vi "Motion_control_X.vi"(0 ".NET Refnum in":refnum<k24>, 1 "maxVelocity":dbl, 2 "acceleration":dbl, 3 "position":dbl) -> (7 ".NET Refnum out":refnum<k24>)   [LabVIEW 2021]
uses:
  C:/Users/User/Documents/Published_files/thorlabs_files/Thorlabs.MotionControl.IntegratedStepperMotorsCLI.dll
  thorlabs_files/Thorlabs.MotionControl.IntegratedStepperMotorsCLI.dll
panel:
  out "end":bool=TRUE
  out "x < y?":bool
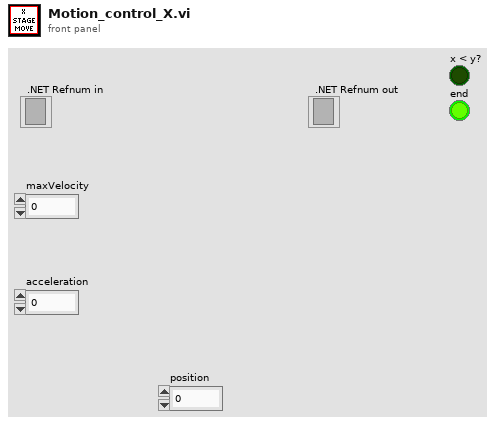
[diagram p1: front panel]
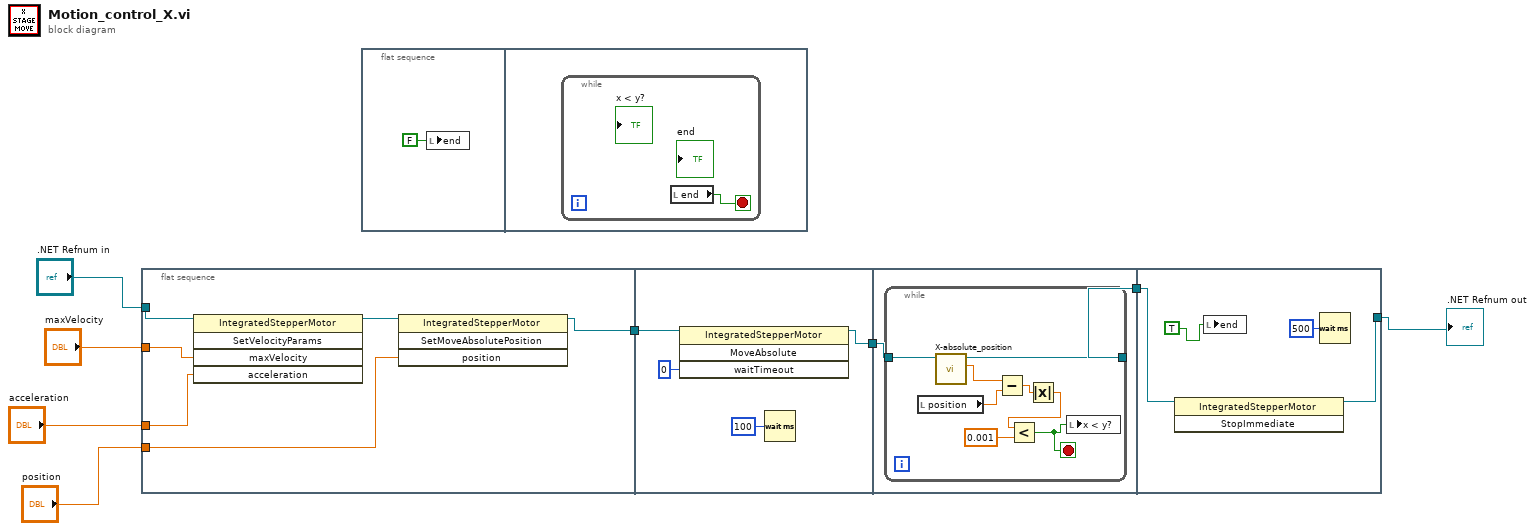
[diagram p0: block diagram]
diagram:
  n1 = flat-sequence {
    tunnel: "maxVelocity" -> [w13]
    tunnel: "acceleration" -> [w12]
    tunnel: ".NET Refnum in" -> [w11]
    tunnel: "position" -> [w10]
    tunnel: [w9] -> w8
    tunnel: w8 -> [w18]
    tunnel: [w16] -> w3
    tunnel: w3 -> [w20]
    tunnel: [w19] -> w2
    tunnel: w2 -> [w30]
    tunnel: [w29] -> w1
    frame #0 {
      n2 = invoke class="IntegratedStepperMotor" method="SetVelocityParams"(reference=w11, "maxVelocity"=w13, "acceleration"=w12) -> (reference out=w14:refnum<k24>)  [unwired: 2 in, 4 out]
      n3 = invoke class="IntegratedStepperMotor" method="SetMoveAbsolutePosition"(reference=w14, "position"=w10) -> (reference out=w9:refnum<k24>)  [unwired: 2 in, 3 out]
    }
    frame #1 {
      n4 = invoke class="IntegratedStepperMotor" method="MoveAbsolute"(reference=w18, "waitTimeout"=0) -> (reference out=w16:refnum<k24>)  [unwired: 2 in, 3 out]
      n5 = Wait (ms)(milliseconds to wait=u32 100) -> ()  [unwired: 1 out]
    }
    frame #2 {
      n6 = while {
        tunnel: w20 -> [w28]
        tunnel: [w25] -> w19
        stop <- w21 stop-if-true
        n7 = local read "position"() -> (w26:dbl)
        n8 = call "X-absolute_position.vi"(".NET Refnum in"=w28) -> ("Numeric"=w27:dbl, ".NET Refnum out"=w25:refnum<k24>)  [unwired: 9 in]
        n9 = Subtract(x=w27, y=w26) -> (x-y=w24:dbl)
        n10 = Absolute Value(x=w24) -> (abs(x)=w23:dbl)
        n11 = Less?(x=w23, y=0.001) -> (x < y?=w21:bool)
        n12 = local write "x < y?"(w21) -> ()
      }
    }
    frame #3 {
      n13 = invoke class="IntegratedStepperMotor" method="StopImmediate"(reference=w30) -> (reference out=w29:refnum<k24>)  [unwired: 2 in, 2 out]
      n14 = local write "end"(TRUE) -> ()
      n15 = Wait (ms)(milliseconds to wait=u32 500) -> ()  [unwired: 1 out]
    }
  }
  n16 = flat-sequence {
    frame #0 {
      n17 = local write "end"(FALSE ("end")) -> ()
    }
    frame #1 {
      n18 = while {
        stop <- w34 stop-if-true
        n19 = local read "end"() -> (w34:bool)
      }
    }
  }
  ".NET Refnum out" <- w1
